vi "LoadPatientDateInfo_Hospital.vi"(8 "error in (no error)":errorcluster, 11 "DataPatientDatePath":path) -> (0 "error out":errorcluster, 3 "hospital":T1)   [LabVIEW 2013, in "main.lvlib"]
uses:
  main.lvlib
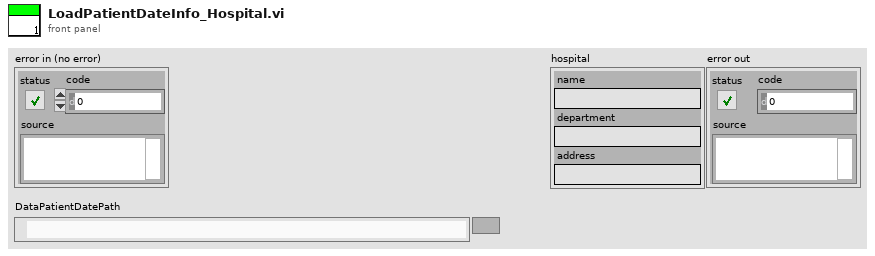
[diagram p1: front panel]
types:
  T1 = cluster{"name":string, "department":string, "address":string}
  T2 = typedef "main.lvlib/date_specific_info.ctl" = cluster{"profile":cluster{"id":string, "name":string, "operator":string, "doctor":string, "comment":string}, "hospital":cluster{"name":string, "department":string, "address":string}, "palpation":cluster{"right":string, "left":string}, "Armpressure Right":cluster{"sys":dbl, "dia":dbl, "puls":dbl, "date":string, "time":string, "code":string, "serial":string, "temp":dbl, "activity":string}[], "Armpressure Left":cluster{"sys":dbl, "dia":dbl, "puls":dbl, "date":string, "time":string, "code":string, "serial":string, "temp":dbl, "activity":string}[]}
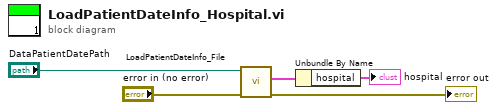
[diagram p0: block diagram]
diagram:
  n1 = call "LoadPatientDateInfo_File.vi"("error in (no error)"="error in (no error)", "DataPatientDatePath"="DataPatientDatePath") -> ("error out"=→"error out":errorcluster, "date_specific_info"=w5:T2)  [unwired: 7 in, 1 out]
  n2 = Unbundle By Name(w5) -> ("hospital"=→"hospital":T1)
